vi "Create_New_Item.vi"(8 "error in (no error)":errorcluster, 11 "Item_Refnums_Array In":T1[](array[typedef])) -> (0 "error out":errorcluster, 3 "Item_Refnums_Array Out":T1[](array[typedef]))   [LabVIEW 2011, in "Root_XControl.xctl"]
uses:
  Root_XControl.xctl
  Controls/References/Item_Refnums.ctl
  Controls/References/Item_Command_Refnum.ctl
  Controls/Item_Command_Enum.ctl
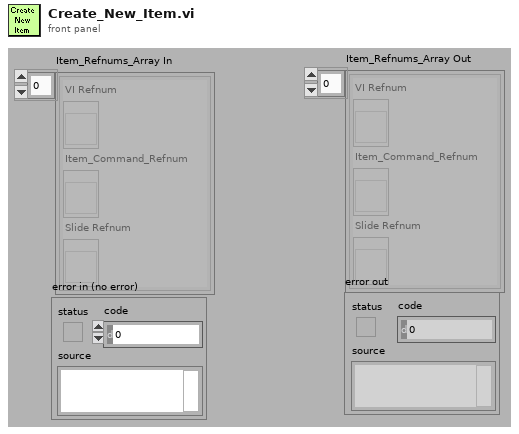
[diagram p1: front panel]
types:
  T1 = typedef "Item_Refnums.ctl" = cluster{"VI Refnum":refnum<vi>, "Item_Command_Refnum":T2, "Slide Refnum":refnum<vi>}
  T2 = typedef "Item_Command_Refnum.ctl" = refnum<vi>
  T3 = enum16{"Always On", "Always Off", "Off While Running"}
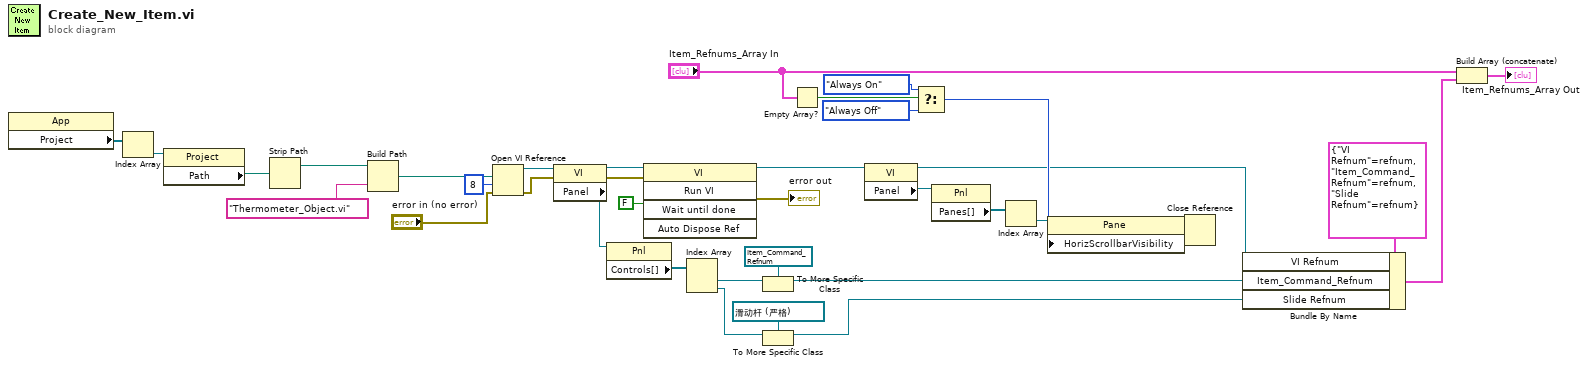
[diagram p0: block diagram]
diagram:
  w24 = FALSE ("Wait Until Done")
  n1 = property class="App"() -> ("Project"=w2:refnum<vi>[])  [unwired: 2 in, 2 out]
  n2 = Index Array(array=w2) -> (element=w1:refnum<vi>)  [unwired: 1 in]
  n3 = property class="Project"(reference=w1) -> ("Path"=w6:path)  [unwired: 1 in, 2 out]
  n4 = Strip Path(path=w6) -> (stripped path=w5:path)  [unwired: 1 out]
  n5 = Build Path(base path=w5, name or relative path="Thermometer_Object.vi") -> (appended path=w3:path)
  n6 = Open VI Reference(vi path=w3, options=8, error in (no error)="error in (no error)") -> (vi reference=w34:refnum<vi>, error out=w35:errorcluster)  [unwired: 3 in]
  n7 = property class="VI"(reference=w34, error in=w35) -> (reference out=w23:refnum<vi>, error out=w22:errorcluster, "Panel"=w33:refnum<vi>)
  n8 = property class="Pnl"(reference=w33) -> ("Controls[]"=w32:refnum<vi>[])  [unwired: 1 in, 2 out]
  n9 = invoke class="VI" method="Run VI"(reference=w23, error in=w22, "Wait until done"=w24, "Auto Dispose Ref"=w24) -> (reference out=w17:refnum<vi>, error out=→"error out":errorcluster)  [unwired: 1 in, 3 out]
  n10 = Index Array(array=w32) -> (element #1=w30:refnum<vi>, element #2=w29:refnum<vi>)  [unwired: 2 in]
  n11 = To More Specific Class(target class=T2 refnum ("Item_Command_Refnum"), reference=w30) -> (specific class reference=w25:T2)  [unwired: 1 in, 1 out]
  n12 = To More Specific Class(target class=refnum<vi> refnum ("Slide Refnum"), reference=w29) -> (specific class reference=w26:refnum<vi>)  [unwired: 1 in, 1 out]
  n13 = Empty Array?(array="Item_Refnums_Array In") -> (empty?=w13:bool)
  n14 = property class="VI"(reference=w17) -> (reference out=w7:refnum<vi>, "Panel"=w16:refnum<vi>)  [unwired: 1 in, 1 out]
  n15 = Select(t=T3."Always On" ("Horizontal Scrollbar Visibility"), s=w13, f=T3."Always Off" ("Horizontal Scrollbar Visibility")) -> (s? t:f=w10:T3)
  n16 = property class="Pnl"(reference=w16) -> ("Panes[]"=w15:refnum<vi>[])  [unwired: 1 in, 2 out]
  n17 = Index Array(array=w15) -> (element=w14:refnum<vi>)  [unwired: 1 in]
  n18 = property class="Pane"(reference=w14, "HorizScrollbarVisibility"=w10) -> (reference out=w8:refnum<vi>, error out=w9:errorcluster)  [unwired: 1 in]
  n19 = Close Reference(reference=w8, error in (no error)=w9) -> ()  [unwired: 1 out]
  n20 = Bundle By Name(cluster=T1 {"VI Refnum"=refnum, "Item_Command_Refnum"=refnum, "Slide Refnum"=refnum} ("Item_Refnums"), "VI Refnum"=w7, "Item_Command_Refnum"=w25, "Slide Refnum"=w26) -> (w21:T1)
  n21 = Build Array (concatenate)("Item_Refnums_Array In", w21) -> (→"Item_Refnums_Array Out":T1[])
